vi "Read incoming label data.vi"(8 "error in (no error)":errorcluster, 10 "From HWIn Buf in":dbl[](array[numeric]), 11 "Label Settings":T1 {"Words"."Param Setting"."Num Bits" min=1 max=32; "Words"."Param Setting"."Start Bit" min=8 max=31; "Words"."Block Data Refs"."Data Reference" format="%.0x"; "Label" format="%.0o"}) -> (0 "error out":errorcluster, 2 "From HWIn Buf out":dbl[](array[numeric]), 3 "Label Settings Out":T1 {"Words"."Param Setting"."Num Bits" min=1 max=32; "Words"."Param Setting"."Start Bit" min=8 max=31; "Words"."Block Data Refs"."Data Reference" format="%.0x"; "Label" format="%.0o"})   [LabVIEW 2016, in "Ballard Arinc-429 Engine.lvlib"]
uses:
  Ballard Arinc-429 Engine.lvlib
  RT Controls/RT Label Settings.ctl
  Shared/Controls and Global/Label.ctl
  Shared/Controls and Global/transferPeriod.ctl
  RT Controls/Driver Data.ctl
  RT Controls/RT Word Settings.ctl
  <vilib>/NI Veristand/Custom Device API/Block Data Reference.ctl
  <vilib>/NI Veristand/Custom Device API/Data Reference.ctl
  RT Controls/RT Param Setting.ctl
  Shared/Controls and Global/Start Bit.ctl
  Shared/Controls and Global/Number of Bits.ctl
  Shared/Controls and Global/TransferType.ctl
  Shared/Ballard Arinc-429 Shared.lvlib
  <vilib>/NI Veristand/Custom Device API/Custom Device API.lvlib
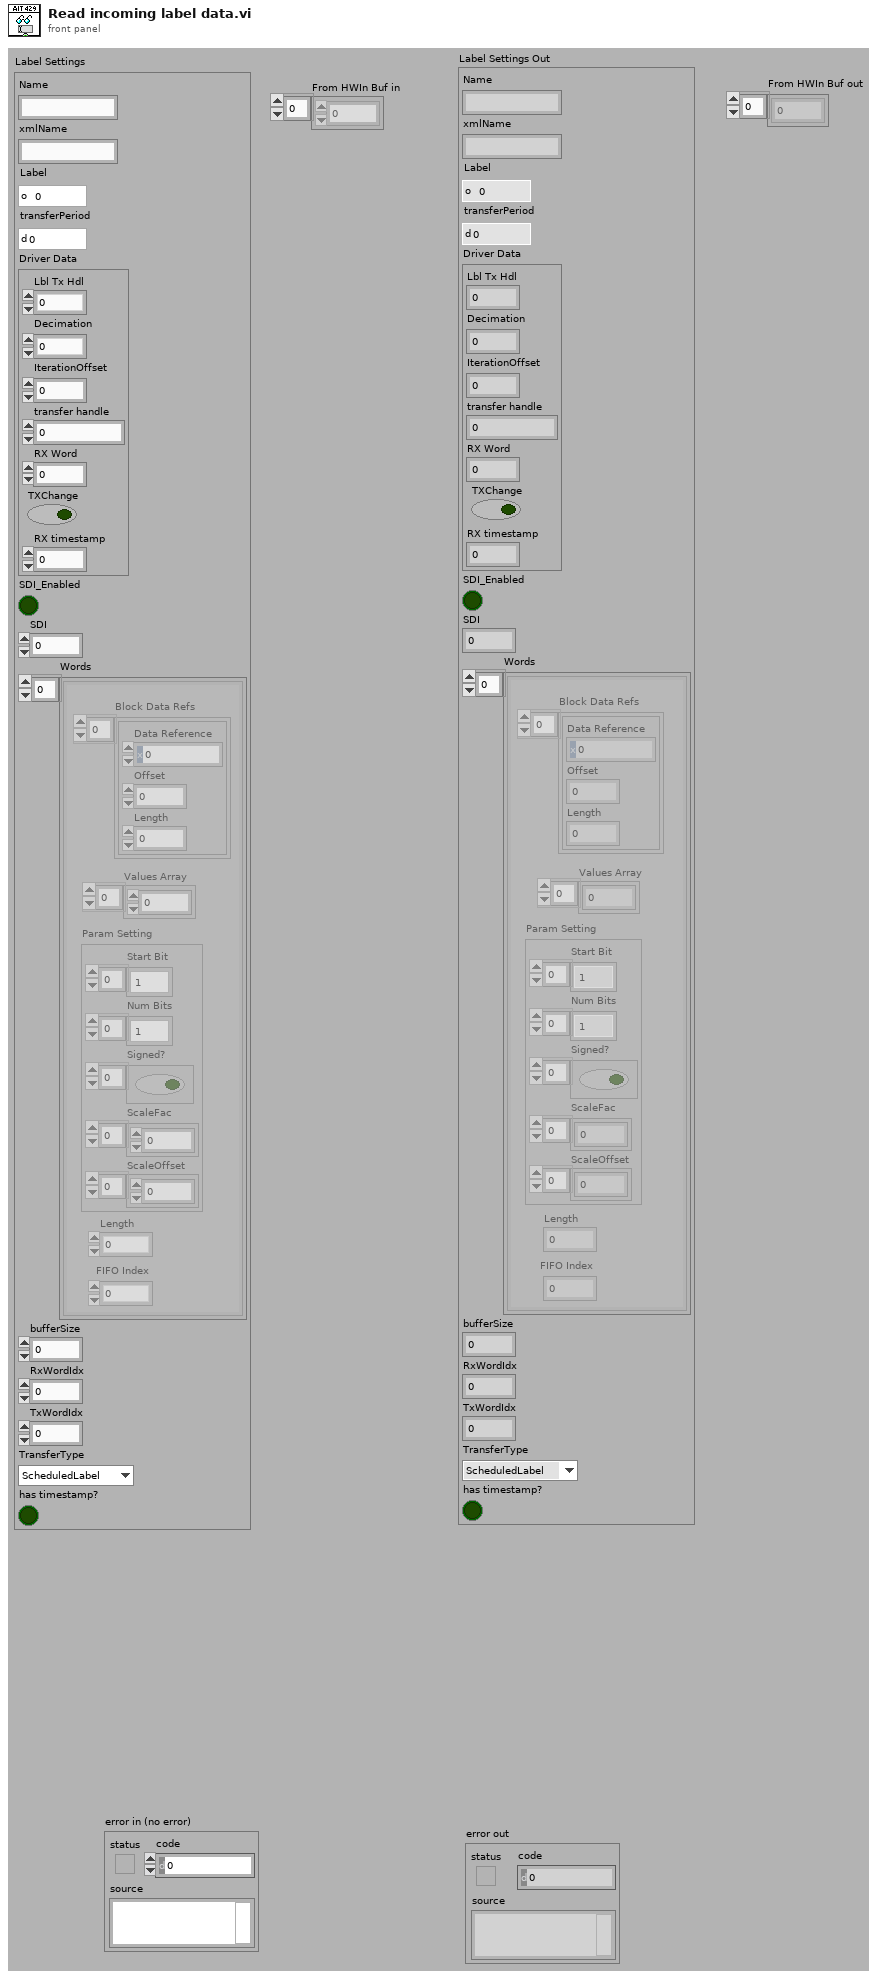
[diagram p1: front panel]
types:
  T1 = typedef "Ballard Arinc-429 Engine.lvlib/RT Label Settings.ctl" = cluster{"Name":string, "xmlName":string, "Label":T2, "transferPeriod":T3, "Driver Data":T4, "SDI_Enabled":bool, "SDI":u8, "Words":T5[], "bufferSize":u32, "RxWordIdx":i32, "TxWordIdx":i32, "TransferType":T11, "has timestamp?":bool}
  T2 = typedef "Ballard Arinc-429 Shared.lvlib/Label.ctl" = u8
  T3 = typedef "Ballard Arinc-429 Shared.lvlib/transferPeriod.ctl" = u32
  T4 = typedef "Ballard Arinc-429 Engine.lvlib/Driver Data.ctl" = cluster{"Lbl Tx Hdl":u32, "Decimation":i32, "IterationOffset":i32, "transfer handle":u32, "RX Word":u32, "TXChange":bool, "RX timestamp":dbl}
  T5 = typedef "Ballard Arinc-429 Engine.lvlib/RT Word Settings.ctl" = cluster{"Block Data Refs":T6[], "Values Array":dbl[], "Length":i32, "FIFO Index":i32, "Param Setting":T8}
  T6 = typedef "Custom Device API.lvlib/Block Data Reference.ctl" = cluster{"Data Reference":T7, "Offset":u64, "Length":u64}
  T7 = typedef "Custom Device API.lvlib/Data Reference.ctl" = i32
  T8 = typedef "Ballard Arinc-429 Engine.lvlib/RT Param Setting.ctl" = cluster{"Start Bit":T9[], "Num Bits":T10[], "Signed?":bool[], "ScaleFac":dbl[], "ScaleOffset":dbl[]}
  T9 = typedef "Ballard Arinc-429 Shared.lvlib/Start Bit.ctl" = i32
  T10 = typedef "Ballard Arinc-429 Shared.lvlib/Number of Bits.ctl" = i32
  T11 = typedef "Ballard Arinc-429 Shared.lvlib/TransferType.ctl" = enum16{"ScheduledLabel", "Acyclic", "Block", "Strobe"}
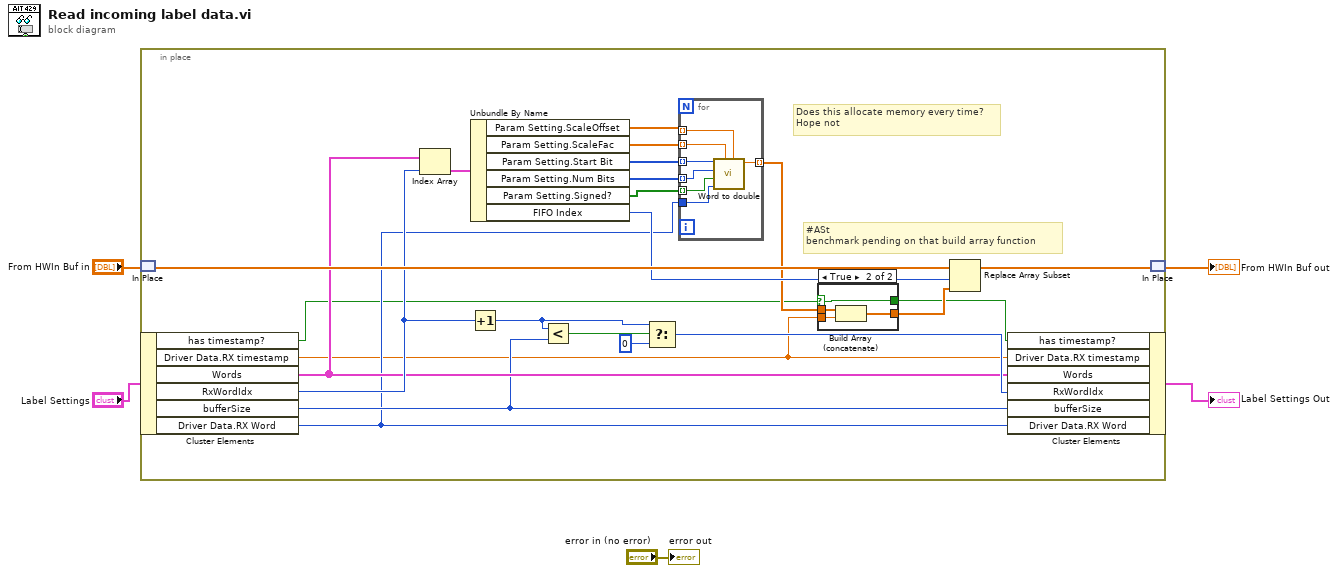
[diagram p0: block diagram]
diagram:
  n1 = in-place {
    # "#ASt\nbenchmark pending on that build array function"
    # "Does this allocate memory every time?\nHope not"
    n2 = in-place-match #1("From HWIn Buf in") -> (w26:dbl[])
    n3 = in-place-cluster #2("Label Settings") -> ("has timestamp?"=w7:bool, "Driver Data.RX timestamp"=w8:dbl, "Words"=w13:T5[], "RxWordIdx"=w24:i32, "bufferSize"=w12:u32, "Driver Data.RX Word"=w11:u32)
    n4 = Index Array(array=w13, index=w24) -> (element=w23:T5)
    n5 = Increment(x=w24) -> (x+1=w14:i32)
    n6 = Unbundle By Name(w23) -> ("Param Setting.ScaleOffset"=w22:dbl[], "Param Setting.ScaleFac"=w21:dbl[], "Param Setting.Start Bit"=w20:T9[], "Param Setting.Num Bits"=w19:T10[], "Param Setting.Signed?"=w18:bool[], "FIFO Index"=w17:i32)
    n7 = Less?(x=w14, y=w12) -> (x < y?=w15:bool)
    n8 = Select(t=w14, s=w15, f=0) -> (s? t:f=w25:i32)
    n9 = for {
      tunnel: [w40] -> w10 mode=indexing
      tunnel: w11 -> [w39]
      tunnel: w18 -> [w38] mode=indexing
      tunnel: w19 -> [w37] mode=indexing
      tunnel: w20 -> [w36] mode=indexing
      tunnel: w21 -> [w35] mode=indexing
      tunnel: w22 -> [w34] mode=indexing
      n10 = call "Word to double.vi"("ScaleOffset (0)"=w34, "ScaleFac (1)"=w35, "word"=w39, "Signed? (F)"=w38, "Number of Bits"=w37, "Start Bit"=w36) -> ("Double"=w40:dbl)  [unwired: 5 in]
    }
    n11 = case shown="True" w7 {
      selector: w7 -> [w28 w30]
      tunnel: w10 -> [w29 w33]
      tunnel: [w29 w32] -> w9
      tunnel: w8 -> [_ w31]
      tunnel: [w28 w30] -> w6
      frame False {
      }
      frame True {
        n12 = Build Array (concatenate)(w33, w31) -> (w32:dbl[])
      }
    }
    n13 = Replace Array Subset(array=w26, new element=w9, index=w17) -> (w27:dbl[])
    n14 = in-place-cluster #2("has timestamp?"=w6, "Driver Data.RX timestamp"=w8, "Words"=w13, "RxWordIdx"=w25, "bufferSize"=w12, "Driver Data.RX Word"=w11) -> (→"Label Settings Out":T1)
    n15 = in-place-match #1(w27) -> (→"From HWIn Buf out":dbl[])
  }
  "error out" <- "error in (no error)"
